vi "Close Device Core.vi"(8 "error in (no error)":errorcluster, 11 "CS++DCPwr in":refnum<class "CS++DCPwr.lvclass">) -> (0 "error out":errorcluster, 3 "CS++DCPwr out":refnum<class "CS++DCPwr.lvclass">)   [LabVIEW 2015, in "CS++DCPwr.lvlib" / "CS++DCPwr.lvclass"]
doc: "Close device driver connection."
uses:
  CS++DCPwr.lvclass
  CSPP_Core/Actors/CS++DeviceActor/CS++DeviceActor.lvclass
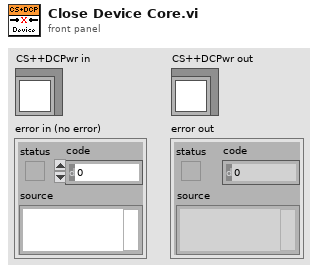
[diagram p1: front panel]
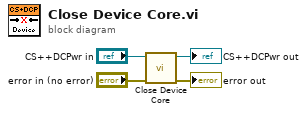
[diagram p0: block diagram]
diagram:
  n1 = call-parent "Close Device Core.vi"("error in (no error)"="error in (no error)", "CS++DeviceActor in"="CS++DCPwr in") -> ("error out"=→"error out":errorcluster, "CS++DeviceActor out"=→"CS++DCPwr out":refnum<class "CS++DCPwr.lvclass">)  [unwired: 8 in]
